vi "Get Logical Datum.vi"(1 "index":i32, 2 "bytestream":refnum<class "Bytestream.lvclass">) -> (0 "datum":T1)   [LabVIEW 2020, in "NI_Bytestream.lvlib" / "Bytestream.lvclass"]
uses:
  <vilib>/Array/Bytestream/Bytestream.lvclass
  <vilib>/Array/Bytestream/Datum.ctl
  <vilib>/Array/Bytestream/Bytestream.lvclass/Bytestream.ctl
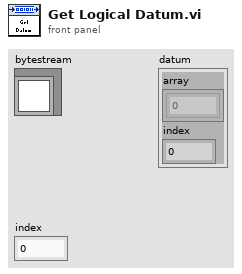
[diagram p1: front panel]
types:
  T1 = typedef "NI_Bytestream.lvlib/Bytestream.lvclass/Datum.ctl" = cluster{"array":u8[], "index":i32}
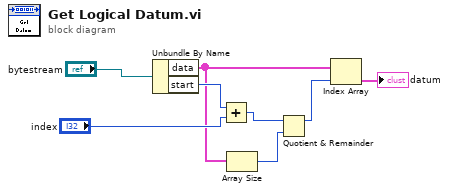
[diagram p0: block diagram]
diagram:
  n1 = Unbundle By Name("bytestream") -> ("data"=w3:T1[], "start"=w7:i32)
  n2 = Add(x=w7, y="index") -> (x+y=w5:i32)
  n3 = Array Size(array=w3) -> (size(s)=w4:i32)
  n4 = Quotient & Remainder(x=w5, y=w4) -> (x-y*floor(x/y)=w2:i32)  [unwired: 1 out]
  n5 = Index Array(array=w3, index=w2) -> (element=→"datum":T1)
